vi "App Version.vi"() -> (2 "App Version":string)   [LabVIEW 2020, in "Volatus.lvlib" / "VolatusAPI.lvclass"]
uses:
  VolatusAPI.lvclass
  VolatusAPI.lvclass/VolatusAPI.ctl
  lv-builder/Builder Core/Builder Core.lvlib
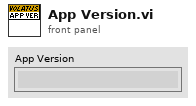
[diagram p1: front panel]
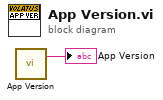
[diagram p0: block diagram]
diagram:
  n1 = call "App Version.vi"() -> ("App Version String"=→"App Version":string)  [unwired: 7 in]
